vi "Insert Calibration Session.vi"(8 "error in (no error)":errorcluster, 10 "Settings in":T1 {"Processing Settings"."Test Parameters"."Allowed Tolerance (%) FS" format="%#_4g"; "Acq Settings"."Config Settings"."Simulated Sensor Injection" scale=0.0..100.0}, 11 "Database":refnum<queue>) -> (0 "error out":errorcluster, 3 "Settings out":T1 {"Processing Settings"."Test Parameters"."Allowed Tolerance (%) FS" format="%#_4g"; "Acq Settings"."Config Settings"."Simulated Sensor Injection" scale=0.0..100.0})   [LabVIEW 2026]
uses:
  controls/UI/Settings Cluster.ctl
  controls/UI/Acq Settings.ctl
  Acquisition/Instrument Specifications Configuration.ctl
  Acquisition/Instrument Specifications Cluster Configuration.ctl
  controls/UI/Measurement Role.ctl
  controls/UI/Config Settings.ctl
  Processing/Processing Settings.ctl
  controls/Messaging Payloads/Sensor CoreData.ctl
  controls/Messaging Payloads/Sensor CoreData Cluster.ctl
  controls/UI/Units Enum.ctl
  controls/UI/Signal Enum.ctl
  Processing/Test Parameters.ctl
  Processing/Test Parameters Cluster.ctl
  controls/UI/Test Sequence Context.ctl
  controls/UI/Test Sequence Context Cluster.ctl
  controls/UI/Direction.ctl
  controls/UI/Session Identfiers.ctl
  controls/UI/Test Sequence Settings.ctl
  controls/UI/Test Sequence State.ctl
  controls/UI/Test Sequence Enum.ctl
  controls/Controller/Stimulus Settings.ctl
  controls/Controller/Stimulus Outputs.ctl
  controls/Controller/Stimulus Output.ctl
  controls/Controller/Controller Core Data.ctl
  controls/Controller/Stimulus Output Configuration.ctl
  controls/Controller/Stimulus Role.ctl
  Architecture/Message Queue/Message Cluster.ctl
  Architecture/Message Queue/Enqueue Message (Single).vi
  Architecture/Message Queue/Message Queue.lvlib
  Settings/Settings.lvlib
  Acquisition/Acquisition.lvlib
  Processing/Processing_Engine.lvlib
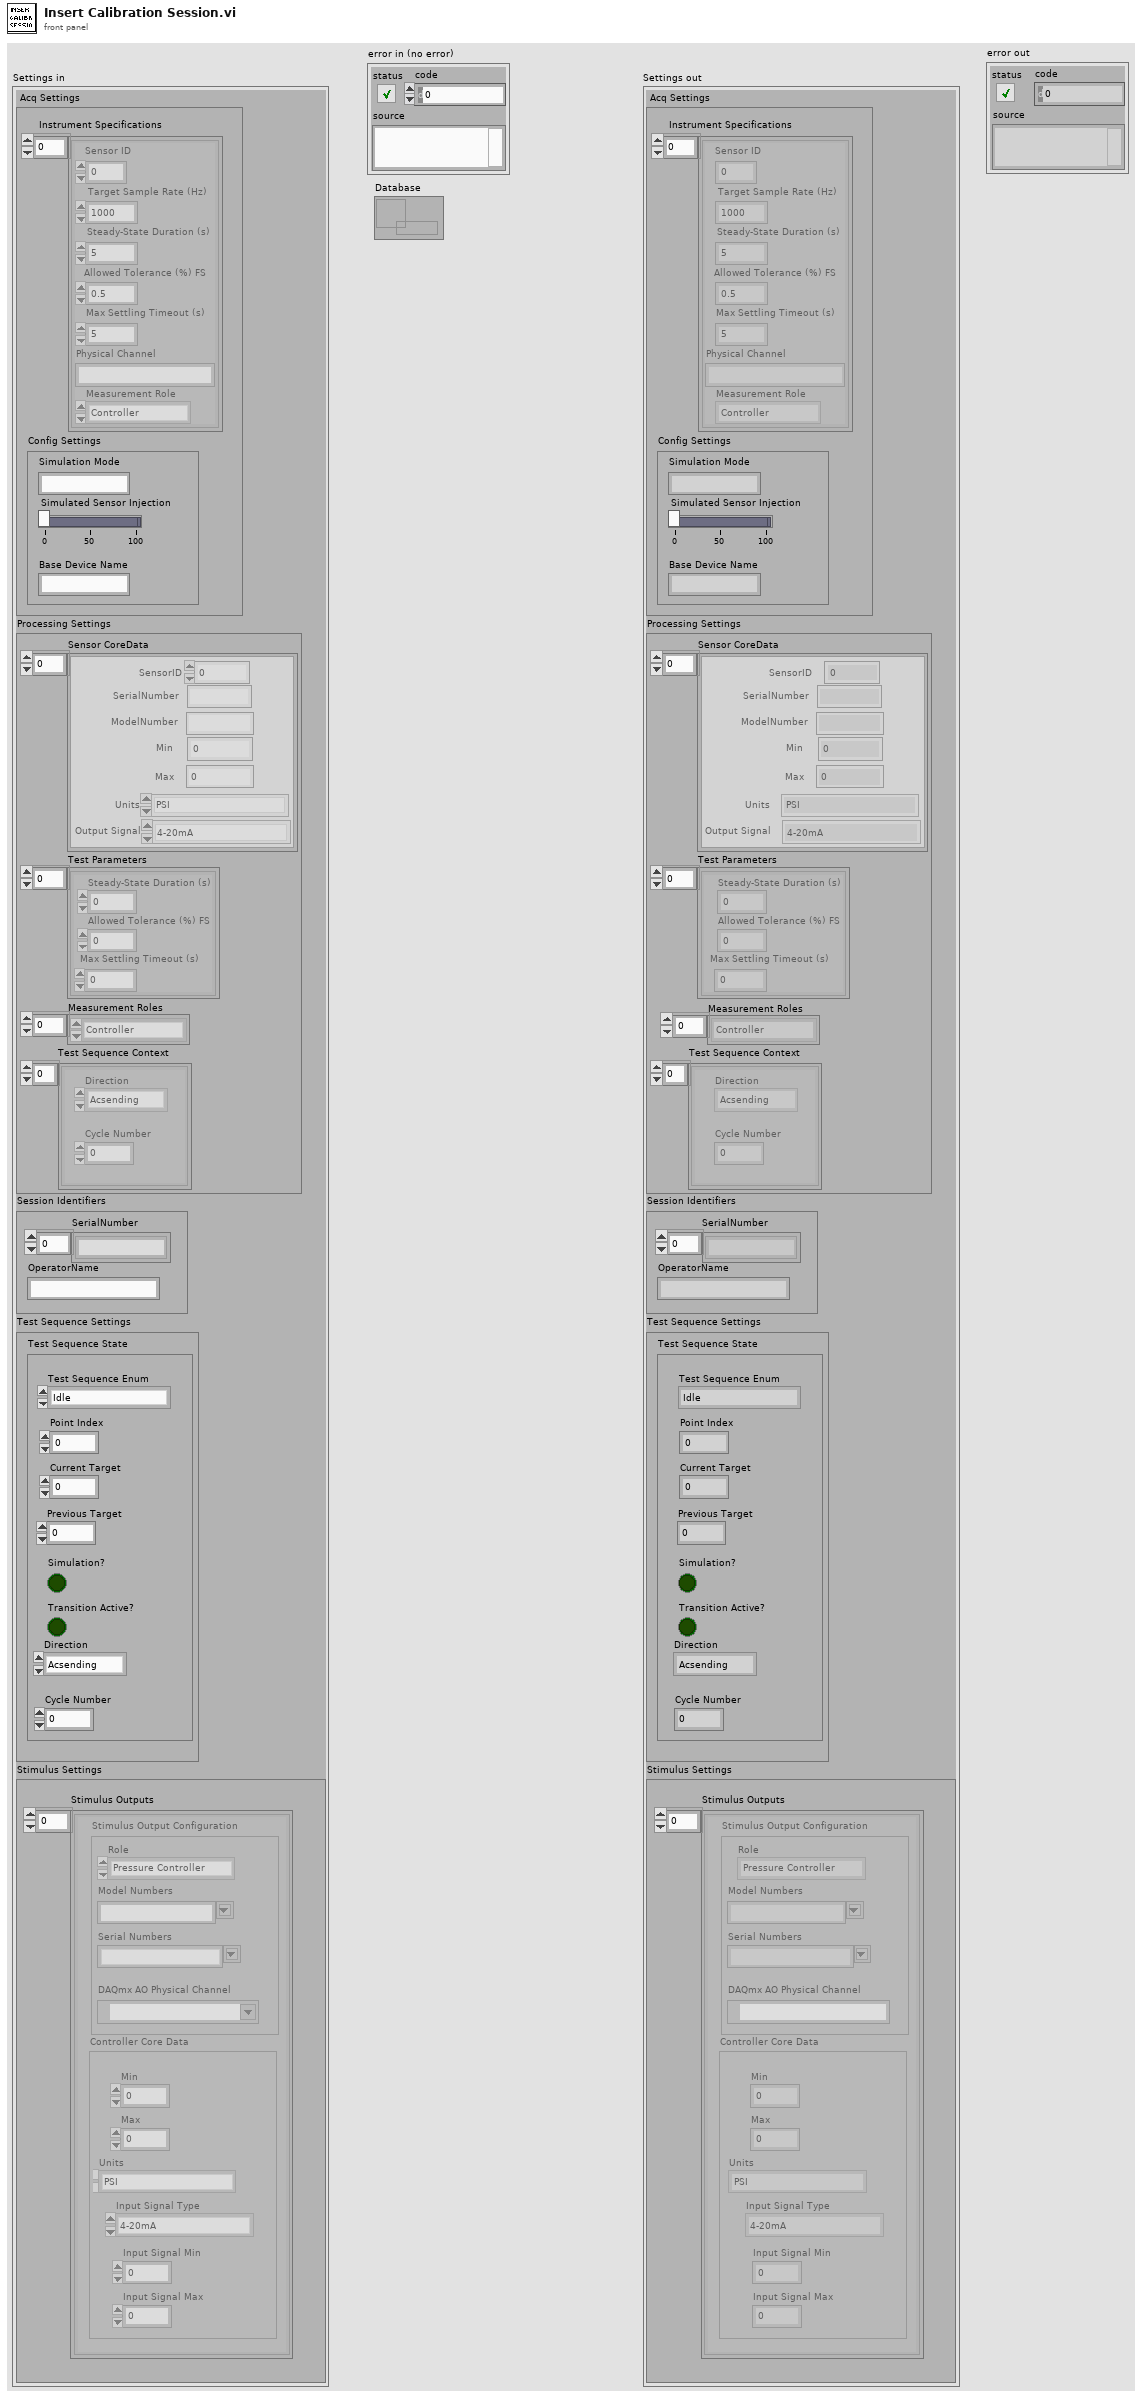
[diagram p1: front panel]
types:
  T1 = typedef "Settings Cluster.ctl" = cluster{"Acq Settings":T2, "Processing Settings":T7, "Session Identifiers":T17, "Test Sequence Settings":T18, "Stimulus Settings":T21}
  T2 = typedef "Acq Settings.ctl" = cluster{"Instrument Specifications":T3, "Config Settings":T6}
  T3 = typedef "Acquisition.lvlib/Instrument Specifications Configuration.ctl" = T4[]
  T4 = typedef "Acquisition.lvlib/Instrument Specifications Cluster Configuration.ctl" = cluster{"Sensor ID":i32, "Target Sample Rate (Hz)":dbl, "Steady-State Duration (s)":i32, "Allowed Tolerance (%) FS":dbl, "Max Settling Timeout (s)":i32, "Physical Channel":string, "Measurement Role":T5}
  T5 = typedef "Settings.lvlib/Measurement Role.ctl" = enum16{"Controller", "Reference", "UUT", "Disable", "All"}
  T6 = typedef "Config Settings.ctl" = cluster{"Simulated Sensor Injection":dbl, "Base Device Name":string, "Simulation Mode":string}
  T7 = typedef "Processing_Engine.lvlib/Processing Settings.ctl" = cluster{"Sensor CoreData":T8, "Test Parameters":T12, "Measurement Roles":T5[], "Test Sequence Context":T14}
  T8 = typedef "Sensor CoreData.ctl" = T9[]
  T9 = typedef "Settings.lvlib/Sensor CoreData Cluster.ctl" = cluster{"SerialNumber":string, "ModelNumber":string, "Min":dbl, "Max":dbl, "Units":T10, "Output Signal":T11, "SensorID":i32}
  T10 = typedef "Units Enum.ctl" = enum16{"PSI", "Deg C", "kPa", "GPM"}
  T11 = typedef "Signal Enum.ctl" = enum16{"4-20mA", "0-10V", "Thermocouple Type K"}
  T12 = typedef "Processing_Engine.lvlib/Test Parameters.ctl" = T13[]
  T13 = typedef "Settings.lvlib/Test Parameters Cluster.ctl" = cluster{"Steady-State Duration (s)":i32, "Allowed Tolerance (%) FS":dbl, "Max Settling Timeout (s)":i32}
  T14 = typedef "Settings.lvlib/Test Sequence Context.ctl" = T15[]
  T15 = typedef "Settings.lvlib/Test Sequence Context Cluster.ctl" = cluster{"Direction":T16, "Cycle Number":i32}
  T16 = typedef "Settings.lvlib/Direction.ctl" = enum16{"Acsending", "Descending"}
  T17 = typedef "Session Identfiers.ctl" = cluster{"SerialNumber":string[], "OperatorName":string}
  T18 = typedef "Test Sequence Settings.ctl" = cluster{"Test Sequence State":T19}
  T19 = typedef "Settings.lvlib/Test Sequence State.ctl" = cluster{"Test Sequence Enum":T20, "Point Index":i32, "Current Target":dbl, "Previous Target":dbl, "Simulation?":bool, "Direction":T16, "Transition Active?":bool, "Cycle Number":i32}
  T20 = typedef "Test Sequence Enum.ctl" = enum16{"Idle", "Start Point", "Point Complete", "Test Complete", "Abort Test", "Reset"}
  T21 = typedef "Settings.lvlib/Stimulus Settings.ctl" = cluster{"Stimulus Outputs":T22}
  T22 = typedef "Settings.lvlib/Stimulus Outputs.ctl" = T23[]
  T23 = typedef "Settings.lvlib/Stimulus Output.ctl" = cluster{"Controller Core Data":T24, "Stimulus Output Configuration":T25}
  T24 = typedef "Settings.lvlib/Controller Core Data.ctl" = cluster{"Min":dbl, "Max":dbl, "Units":T10, "Input Signal Type":T11, "Input Signal Min":dbl, "Input Signal Max":dbl}
  T25 = typedef "Settings.lvlib/Stimulus Output Configuration.ctl" = cluster{"DAQmx AO Physical Channel":tag, "Role":T26, "Model Numbers":string, "Serial Numbers":string}
  T26 = typedef "Stimulus Role.ctl" = enum16{"Pressure Controller", "Temperature Controller"}
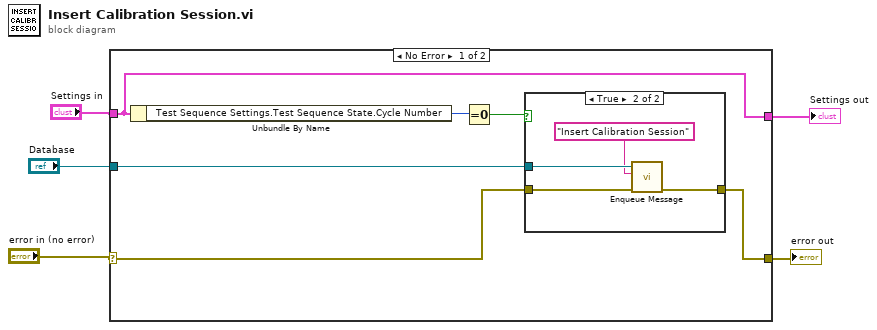
[diagram p0: block diagram]
diagram:
  n1 = case shown="No Error" "error in (no error)" {
    selector: "error in (no error)" -> [w10 w18]
    tunnel: "Settings in" -> [w6 w17]
    tunnel: [w9 w18] -> w3
    tunnel: "Database" -> [w11 _]
    tunnel: [w6 w17] -> w1
    frame No Error {
      n2 = Unbundle By Name(w6) -> ("Test Sequence Settings.Test Sequence State.Cycle Number"=w8:i32)
      n3 = Equal To 0?(x=w8) -> (x = 0?=w7:bool)
      n4 = case shown="True" w7 {
        tunnel: w11 -> [_ w16]
        tunnel: w10 -> [w12 w14]
        tunnel: [w12 w13] -> w9
        frame False {
        }
        frame True {
          n5 = call-poly "Enqueue Message.vi"("error in (no error)"=w14, "Message"="Insert Calibration Session", "Message Queue"=w16) -> ("error out"=w13:errorcluster)  [unwired: 7 in, 1 out]
        }
      }
    }
    frame Error {
    }
  }
  "error out" <- w3
  "Settings out" <- w1
